vi "Fake Passing Test.vi"() -> ()   [LabVIEW 2017, in "LVUnit Test Executor.Tests.lvlib"]
uses:
  LVUnit Test Executor.Tests.lvlib
panel:
  out "error out":errorcluster
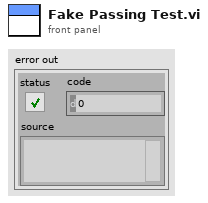
[diagram p1: front panel]
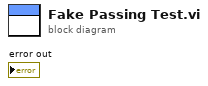
[diagram p0: block diagram]
diagram:
